vi "GetSingleAnalogInputVal.vi"(8 "error in (no error)":errorcluster, 10 "Pin number 0-7":dbl, 11 "SerialPortRef":T1) -> (0 "error out":errorcluster, 1 "Scaled Voltage":dbl, 2 "Raw Voltage":u32, 3 "SerialPortRef 2":T1)   [LabVIEW 2015]
uses:
  <vilib>/Rock Robotics/WPI/SerialPort/WPI_SerialPortRef.ctl
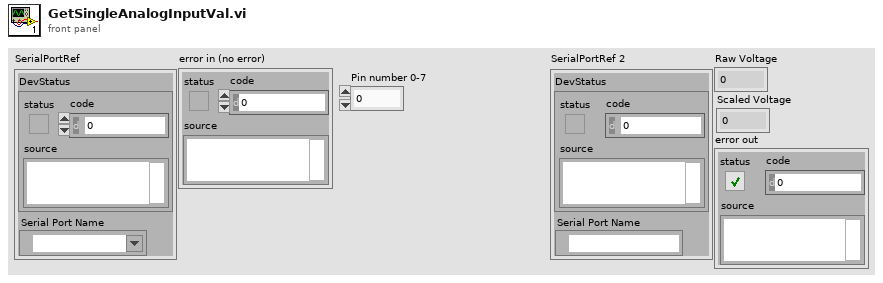
[diagram p1: front panel]
types:
  T1 = typedef "WPI_SerialPortRef.ctl" = cluster{"DevStatus":errorcluster, "Serial Port Name":refnum<visa-resource-name>}
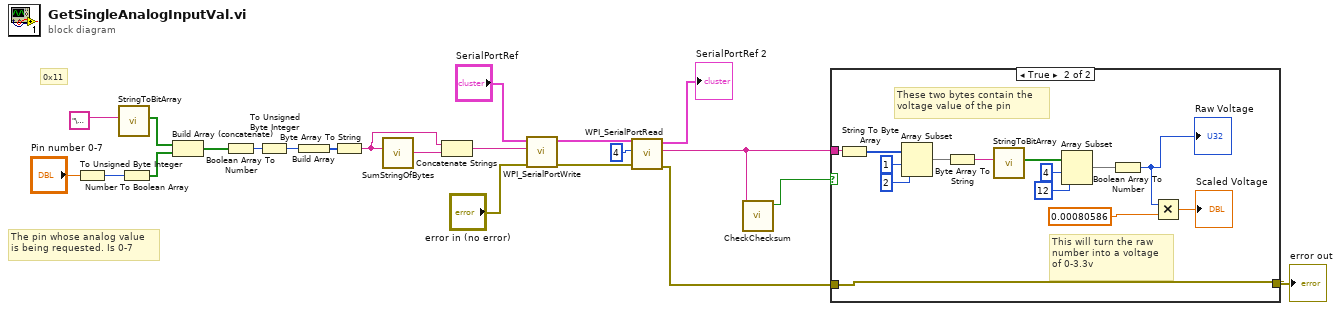
[diagram p0: block diagram]
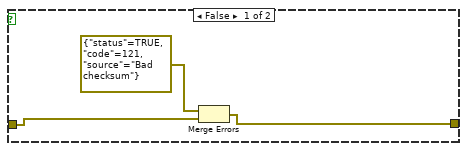
[diagram p2: hidden frame]
diagram:
  # "The pin whose analog value\nis being requested. Is 0-7"
  # "0x11"
  n1 = To Unsigned Byte Integer(number="Pin number 0-7") -> (unsigned 8bit integer=w12:u8)
  n2 = call "StringToBitArray.vi"("string"="\u0011" ("Buffer")) -> ("Array"=w9:bool[])  [unwired: 10 in]
  n3 = Number To Boolean Array(number=w12) -> (Boolean array=w8:bool[])
  n4 = Build Array (concatenate)(w9, w8) -> (w7:bool[])
  n5 = Boolean Array To Number(Boolean array=w7) -> (number=w4:u32)
  n6 = To Unsigned Byte Integer(number=w4) -> (unsigned 8bit integer=w6:u8)
  n7 = Build Array(w6) -> (w5:u8[])
  n8 = Byte Array To String(unsigned byte array=w5) -> (string=w3:string)
  n9 = call "SumStringOfBytes.vi"("String Of Bytes"=w3) -> ("SumAsString"=w2:string)  [unwired: 10 in]
  n10 = Concatenate Strings(w3, w2) -> (w1:string)
  n11 = call <vilib>:"WPI_SerialPortWrite.vi"("error in (no error)"="error in (no error)", "Buffer"=w1, "SerialPortRef"="SerialPortRef") -> ("error out"=w18:errorcluster, "SerialPortRef"=w22:T1)  [unwired: 6 in, 1 out]
  n12 = call <vilib>:"WPI_SerialPortRead.vi"("error in (no error)"=w18, "Num Bytes to Read"=u32 4, "SerialPortRef"=w22) -> ("error out"=w13:errorcluster, "Buffer"=w16:string, "SerialPortRef"=→"SerialPortRef 2":T1)  [unwired: 6 in]
  n13 = call "CheckChecksum.vi"("String"=w16) -> ("x = y?"=w15:bool)  [unwired: 10 in]
  n14 = case shown="True" w15 {
    tunnel: w16 -> [_ w27]
    tunnel: w13 -> [w25 w26]
    tunnel: [w23 w26] -> w14
    frame False {
      n15 = Merge Errors(errorcluster {"status"=TRUE, "code"=121, "source"="Bad checksum"} ("error in"), w25) -> (w23:errorcluster)
    }
    frame True {
      # "This will turn the raw \nnumber into a voltage \nof 0-3.3v"
      # "These two bytes contain the \nvoltage value of the pin"
      n16 = String To Byte Array(string=w27) -> (unsigned byte array=w39:u8[])
      n17 = Array Subset(array=w39, index=1, length=2) -> (w36:u8[])
      n18 = Byte Array To String(unsigned byte array=w36) -> (string=w35:string)
      n19 = call "StringToBitArray.vi"("string"=w35) -> ("Array"=w34:bool[])  [unwired: 10 in]
      n20 = Array Subset(array=w34, index=4, length=12) -> (w31:bool[])
      n21 = Boolean Array To Number(Boolean array=w31) -> (number=w30:u32)
      "Raw Voltage" <- w30
      n22 = Multiply(x=w30, y=0.00080586) -> (x*y=→"Scaled Voltage":dbl)
    }
  }
  "error out" <- w14
